vi "Archivos en hojas de calculo.vi"() -> ()   [LabVIEW 2020]
uses:
  <vilib>/Analysis/NI_AALBase.lvlib
panel:
  out "Tabla":string[][](array[string])
  out "Waveform Graph":dbl[][](graph)
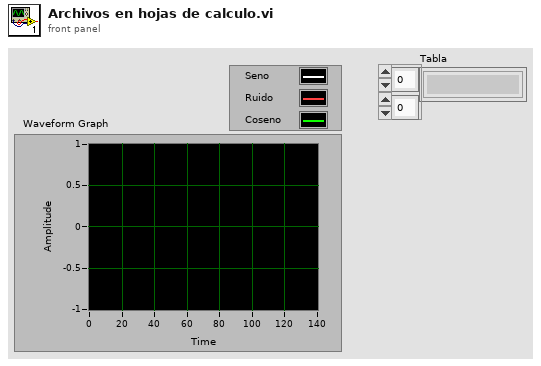
[diagram p1: front panel]
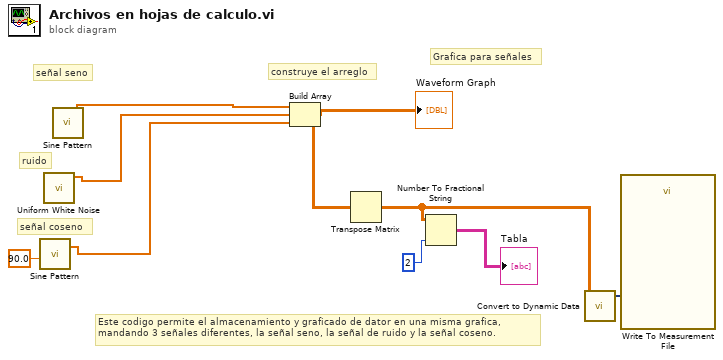
[diagram p0: block diagram]
diagram:
  # "construye el arreglo"
  # "Grafica para señales"
  # "señal coseno"
  # "ruido"
  # "señal seno"
  # "Este codigo permite el almacenamiento y graficado de dator en una misma grafica, \nmandando 3 señales diferentes, la señal seno, la señal de ruido y la señal coseno."
  n1 = call <vilib>:"Sine Pattern.vi"("phase(degrees)"=90.0) -> ("Sinusoidal Pattern"=w2:dbl[])  [unwired: 3 in, 1 out]
  n2 = call <vilib>:"Uniform White Noise.vi"() -> ("uniform white noise"=w4:dbl[])  [unwired: 10 in, 1 out]
  n3 = call <vilib>:"Sine Pattern.vi"() -> ("Sinusoidal Pattern"=w9:dbl[])  [unwired: 4 in, 1 out]
  n4 = Build Array(w9, w4, w2) -> (w1:dbl[][])
  "Waveform Graph" <- w1
  n5 = Transpose Matrix(1:w1) -> (0:w6:dbl[][])
  n6 = Number To Fractional String(number=w6, precision (6)=2) -> (F-format string=→"Tabla":string[][])  [unwired: 2 in]
  n7 = call "Convert to Dynamic Data"("2D Array"=w6) -> ("Dynamic Data Type"=w5:dynamicdata)  [unwired: 3 in]
  n8 = call "Write To Measurement File"("Signals"=w5) -> ()  [unwired: 16 in, 3 out]
